vi "Message_BoxA.vi"(1 "Texte":string, 5 "Modale (T)":bool=TRUE, 6 "Error In":errorcluster, 7 "Titre":string, 8 "Défaut":u8=1 min=1 max=4, 9 "Bouton":T3(ring), 10 "Type":T1(ring)) -> (0 "Error Out":errorcluster, 3 "Bouton pressé":T2(ring))   [LabVIEW 2018]
doc: "Appel d'une boîte de dialogue. La fonction originale provient du cours Advanced I.\n\n\nDéfaut : numéro du bouton par défaut\n\nType : type de boîte de dialogue\n\nBouton : bouton(s) de la boîte\n\nTitre : texte à afficher dans la barre de titre\n\nTexte : texte à afficher dans la boîte de dialogue\n\nModale : action de la boîte de dialogue tant que l'utilisateur n'a pas répondu\n - False (Application) : l'application est interrompue\n - True (Système) : toutes les applications sont interrompues\n\n\nBouton pressé : bouton qui a été pressé\n\n\nJ. Bögli Sonceboz SA\nJuin 2002"
uses:
  USER32.DLL
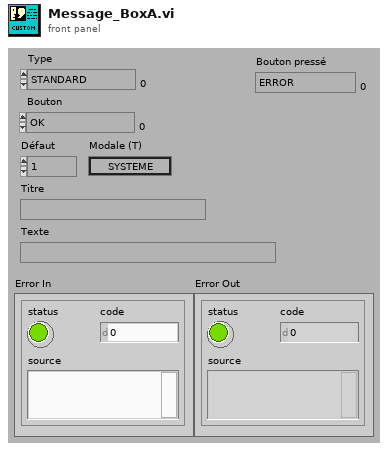
[diagram p1: front panel]
types:
  T1 = enum8{"STANDARD", "CRITICAL", "QUESTION", "EXCLAMATION", "INFORMATION"}
  T2 = enum16{"ERROR", "OK", "CANCEL", "ABORT", "RETRY", "IGNORE", "YES", "NO"}
  T3 = enum8{"OK", "OK CANCEL", "ABORT RETRY IGNORE", "YES NO CANCEL", "YES NO", "RETRY CANCEL"}
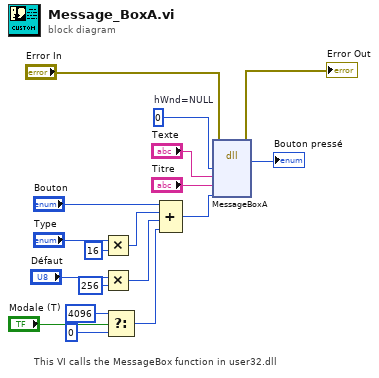
[diagram p0: block diagram]
diagram:
  w17 = 0  # hWnd=NULL
  # "This VI calls the MessageBox function in user32.dll"
  n1 = Multiply(x="Type", y=u32 16) -> (x*y=w12:u32)
  n2 = Multiply(x="Défaut", y=u32 256) -> (x*y=w8:u32)
  n3 = Select(t=u32 4096, s="Modale (T)", f=u32 0) -> (s? t:f=w3:u32)
  n4 = Compound Arithmetic op=ADD("Bouton", w12, w8, w3) -> (w11:u32)
  n5 = dll-call lib="USER32.DLL" fn="MessageBoxA"(error in="Error In", "hWnd"=w17, "lpText"="Texte", "lpCaption"="Titre", "uType"=w11) -> (error out=→"Error Out":errorcluster, →"Bouton pressé":i32)  [unwired: 6 in, 1 out]
